vi "changeRange.vi"(8 "error in (no error)":errorcluster, 9 "Input Range":dbl=10.0 format="%#_10g", 10 "ElectrometerController in":refnum<class "ElectrometerController.lvclass">, 11 "ReadyState in":refnum<class "ReadyState.lvclass">) -> (0 "error out":errorcluster, 2 "ElectrometerController out":refnum<class "ElectrometerController.lvclass">, 3 "ReadyState out":refnum<class "ReadyState.lvclass">)   [LabVIEW 2016, in "ReadyState.lvclass"]
uses:
  ReadyState.lvclass
  ElectrometerController/ElectrometerController.lvclass
  ts_electrometeruserevents/Typedefs/StateValue.ctl
  ts_electrometeruserevents/Typedefs/PubDataSV.ctl
  ts_sallv_calibrationelectrometer/DataTypes/logevent_measureRange.ctl
  ts_electrometeruserevents/Typedefs/CommandValue.ctl
  ElectrometerController/ElectrometerController.lvclass/ElectrometerController.ctl
  ts_electrometeruserevents/PubSubDataEvent/PubSubDataEvent.lvclass
  Electrometer.lvclass
  ElectrometerConfiguration/ElectrometerInternalConfiguration.lvclass
  ts_electrometeruserevents/Typedefs/ElectrometerTypedefs.lvlib
  ts_sallv_calibrationelectrometer/SALLV_calibrationElectrometer.lvlib
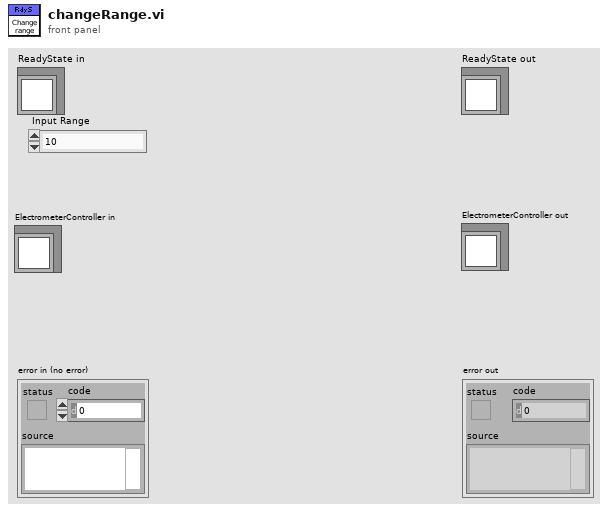
[diagram p1: front panel]
types:
  T1 = typedef "ElectrometerTypedefs.lvlib/CommandValue.ctl" = enum16{"ClearError", "Disable", "Enable", "Exit", "GoToStandby", "OnHeartbeat", "OnIncomingMessagingError", "OnInterrupt", "Start", "SetDigitalFilter", "StartScan", "StartScanDt", "StartScanReachIntensity", "StopScan", "SetIntegrationTime", "PerformZeroCalib", "SetRange", "SetMode", "Power"}
  T2 = cluster{"appliedSettingsMatchStart":bool, "Timestamp":dbl}
  T3 = typedef "ElectrometerTypedefs.lvlib/PubDataSV.ctl" = enum16{"DetailedState", "ErrorCode", "Heartbeat", "LoopTime_ms", "LoopTimeOutOfRange", "RejectedCommand", "SummaryState", "Timestamp", "SettingVersions", "SettingsAppliedSerialConfiguration", "AppliedSettingsMatchStart", "InternalState", "Intensity", "MeasureType", "MeasureRange", "DigitalFilterChange", "IntensityReq", "IntegrationTime", "SettingsAppliedReadingSettings"}
  T4 = typedef "SALLV_calibrationElectrometer.lvlib/logevent_measureRange.ctl" = cluster{"rangeValue":sgl, "electId":i16, "priority":i32}
  T5 = typedef "ElectrometerTypedefs.lvlib/StateValue.ctl" = enum16{"", "DisabledState", "EnabledState", "FaultState", "OffState", "StandbyState", "ReadyState", "ConfiguringState", "ManualReadingState", "UntilIntensityReadingState", "SetDurationReadingState", "BufferReadingState"}
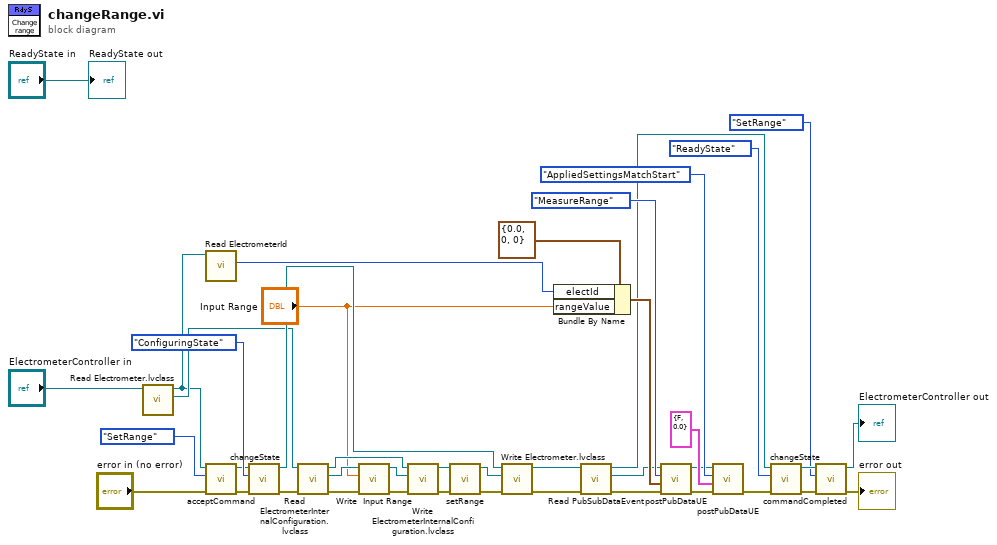
[diagram p0: block diagram]
diagram:
  n1 = call-dynamic "Read Electrometer.lvclass.vi"("ElectrometerController in"="ElectrometerController in") -> ("Electrometer.lvclass"=w28:refnum<class "Electrometer.lvclass">, "ElectrometerController out"=w10:refnum<class "ElectrometerController.lvclass">)  [unwired: 8 in, 1 out]
  n2 = call-dynamic "Read ElectrometerId.vi"("ElectrometerController in"=w10) -> ("ElectrometerId"=w16:enum16{"", "ID1", "ID2"})  [unwired: 8 in, 2 out]
  n3 = call "acceptCommand.vi"("error in (no error)"="error in (no error)", "CommandValue"=CommandValue."SetRange", "ElectrometerController in"=w10) -> ("error out"=w8:errorcluster, "ElectrometerController out"=w9:refnum<class "ElectrometerController.lvclass">)  [unwired: 7 in]
  n4 = call "changeState.vi"("error in (no error)"=w8, "StateValue"=StateValue."ConfiguringState", "ElectrometerController in"=w9) -> ("error out"=w27:errorcluster, "ElectrometerController out"=w29:refnum<class "ElectrometerController.lvclass">)  [unwired: 7 in]
  n5 = call-dynamic "Read ElectrometerInternalConfiguration.lvclass.vi"("error in (no error)"=w27, "Electrometer in"=w28) -> ("error out"=w34:errorcluster, "ElectrometerInternalConfiguration.lvclass"=w37:refnum<class "ElectrometerInternalConfiguration.lvclass">, "Electrometer out"=w33:refnum<class "Electrometer.lvclass">)  [unwired: 7 in]
  n6 = call-dynamic "Write  Input Range .vi"("error in (no error)"=w34, "Input Range"="Input Range", "ElectrometerInternalConfiguration in"=w37) -> ("error out"=w35:errorcluster, "ElectrometerInternalConfiguration out"=w36:refnum<class "ElectrometerInternalConfiguration.lvclass">)  [unwired: 7 in]
  n7 = call-dynamic "Write ElectrometerInternalConfiguration.lvclass.vi"("error in (no error)"=w35, "ElectrometerInternalConfiguration.lvclass"=w36, "Electrometer in"=w33) -> ("error out"=w32:errorcluster, "Electrometer out"=w26:refnum<class "Electrometer.lvclass">)  [unwired: 7 in]
  n8 = call "setRange.vi"("error in (no error)"=w32, "Electrometer in"=w26) -> ("error out"=w31:errorcluster, "Electrometer out"=w30:refnum<class "Electrometer.lvclass">)  [unwired: 8 in]
  n9 = call-dynamic "Write Electrometer.lvclass.vi"("error in (no error)"=w31, "Electrometer.lvclass"=w30, "ElectrometerController in"=w29) -> ("error out"=w15:errorcluster, "ElectrometerController out"=w13:refnum<class "ElectrometerController.lvclass">)  [unwired: 7 in]
  n10 = Bundle By Name(cluster=T4 {"rangeValue"=0.0, "electId"=0, "priority"=0} ("logevent_measureRange"), "electId"=w16, "rangeValue"="Input Range") -> (w23:T4)
  n11 = call "Read PubSubDataEvent.vi"("error in (no error)"=w15, "ElectrometerController in"=w13) -> ("error out"=w14:errorcluster, "PubSubDataEvent.lvclass"=w11:refnum<class "PubSubDataEvent.lvclass">, "ElectrometerController out"=w12:refnum<class "ElectrometerController.lvclass">)  [unwired: 7 in]
  n12 = call "postPubDataUE.vi"("error in (no error)"=w14, "value"=w23, "pubDataSV"=PubDataSV."MeasureRange", "PubSubDataEvent in"=w11) -> ("error out"=w20:errorcluster, "PubSubDataEvent out"=w18:refnum<class "PubSubDataEvent.lvclass">)  [unwired: 6 in]
  n13 = call "postPubDataUE.vi"("error in (no error)"=w20, "value"=T2 {"appliedSettingsMatchStart"=FALSE, "Timestamp"=0.0} ("event data"), "pubDataSV"=PubDataSV."AppliedSettingsMatchStart", "PubSubDataEvent in"=w18) -> ("error out"=w19:errorcluster)  [unwired: 6 in, 1 out]
  n14 = call "changeState.vi"("error in (no error)"=w19, "StateValue"=StateValue."ReadyState", "ElectrometerController in"=w12) -> ("error out"=w5:errorcluster, "ElectrometerController out"=w6:refnum<class "ElectrometerController.lvclass">)  [unwired: 7 in]
  n15 = call "commandCompleted.vi"("error in (no error)"=w5, "CommandValue"=CommandValue."SetRange", "ElectrometerController in"=w6) -> ("error out"=→"error out":errorcluster, "ElectrometerController out"=→"ElectrometerController out":refnum<class "ElectrometerController.lvclass">)  [unwired: 7 in]
  "ReadyState out" <- "ReadyState in"
